vi "array.vi"() -> ()   [LabVIEW 2016]
panel:
  out "number (0 to 1)":dbl
  out "Array":dbl[](array[numeric])
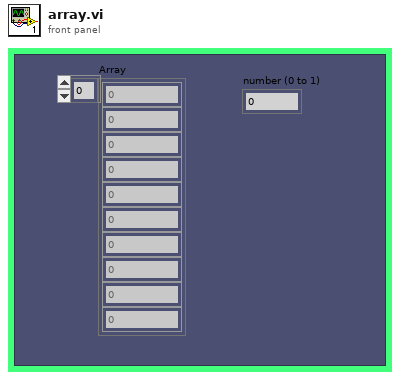
[diagram p1: front panel]
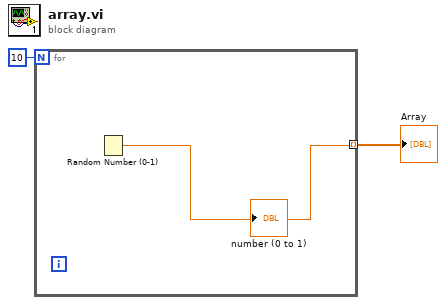
[diagram p0: block diagram]
diagram:
  n1 = for {
    N: 10 -> [_]
    tunnel: [w3] -> w2 mode=indexing
    n2 = Random Number (0-1)() -> (number: 0 to 1=w3:dbl)
    "number (0 to 1)" <- w3
  }
  "Array" <- w2
